vi "DynPid_filtered.vi"() -> ()   [LabVIEW 2019]
uses:
  <vilib>/Analysis/Matrix/Datatypes/RealMatrix.ctl
  <vilib>/userDefined/High Color/IMAQdx.ctl
  <vilib>/Platform/TimedLoop/XDataNode/timing_clust.ctl
  <vilib>/Platform/TimedLoop/XDataNode/nitl_modes.ctl
  <vilib>/Platform/TimedLoop/XDataNode/wakeup.ctl
  <vilib>/myRIO/Instrument Drivers/Onboard IO/AO/typedefs/AO Reference.ctl
  <vilib>/myRIO/Common/Instrument Driver Framework/Utilities/typedefs/myRIO Generic Hardware Reference.ctl
  <vilib>/myRIO/Common/Instrument Driver Framework/Utilities/typedefs/Hardware Version Enum.ctl
  <vilib>/myRIO/Common/Instrument Driver Framework/Utilities/typedefs/myRIO v1.0 Reference.ctl
  <vilib>/myRIO/Common/Instrument Driver Framework/Utilities/typedefs/Generic FPGA Reference.ctl
  <vilib>/myRIO/Common/Instrument Driver Framework/myRIO v1.0/AO/typedefs/AO Channels List.ctl
  <vilib>/myRIO/Common/Instrument Driver Framework/myRIO v1.0/AO/typedefs/AO Channels Enum.ctl
  <vilib>/myRIO/Common/Instrument Driver Framework/Utilities/typedefs/Analog Scaling Constants List.ctl
  <vilib>/myRIO/Common/Instrument Driver Framework/Utilities/typedefs/Analog Scaling Constants.ctl
  <vilib>/userDefined/High Color/nirio_resource_hc.ctl
  <vilib>/myRIO/Common/Instrument Driver Framework/myRIO v1.0/Encoder/typedefs/Encoder Signal Mode.ctl
  <vilib>/myRIO/Instrument Drivers/Onboard IO/Encoder/typedefs/Encoder Reference.ctl
  <vilib>/myRIO/Common/Instrument Driver Framework/myRIO v1.0/Encoder/typedefs/Encoder Channels Enum.ctl
  <vilib>/myRIO/Common/Instrument Driver Framework/myRIO v1.0/Encoder/typedefs/Encoder Configuration v1.0.ctl
  <vilib>/myRIO/Common/Instrument Driver Framework/Utilities/vis/Is FPGA Ref Available.vi
  <vilib>/myRIO/Common/Instrument Driver Framework/myRIO v1.0/AO/vis/myRIO v1.1 Open AO.vi
  <vilib>/myRIO/Instrument Drivers/Onboard IO/AO/vis/Write.vi
  <vilib>/myRIO/Common/Instrument Driver Framework/myRIO v1.0/Encoder/vis/myRIO v1.1 Open Encoder.vi
  <vilib>/myRIO/Instrument Drivers/Onboard IO/Encoder/vis/Read.vi
  <vilib>/myRIO/Common/Instrument Driver Framework/Utilities/vis/Validate Channels.vi
  <vilib>/myRIO/Common/Instrument Driver Framework/myRIO v1.0/AO/vis/myRIO v1.0 Reserve AO.vi
  <vilib>/myRIO/Common/Instrument Driver Framework/myRIO v1.0/Encoder/vis/myRIO v1.0 Reserve Encoder.vi
  <vilib>/Analysis/baseanly.llb/A x B.vi
  <vilib>/Analysis/baseanly.llb/A x Vector.vi
  <vilib>/myRIO/Common/Instrument Driver Framework/myRIO v1.0/AO/vis/myRIO v1.0 Build MUX Configuration AO.vi
  <vilib>/myRIO/Common/Instrument Driver Framework/myRIO v1.0/Resource Manager/vis/myRIO v1.0 Reserve Channel List.vi
  <vilib>/myRIO/Common/Instrument Driver Framework/myRIO v1.0/Encoder/vis/myRIO v1.0 Build MUX Configuration Encoder.vi
  <vilib>/myRIO/Common/Instrument Driver Framework/myRIO v1.0/Resource Manager/vis/myRIO v1.0 Reserve Channel.vi
  <vilib>/myRIO/Common/Instrument Driver Framework/myRIO v1.0/Resource Manager/vis/myRIO v1.0 Unreserve Channel.vi
  <vilib>/myRIO/Common/Instrument Driver Framework/myRIO v1.0/Resource Manager/vis/myRIO v1.0 Create Configuration List.vi
  <vilib>/myRIO/Common/Instrument Driver Framework/myRIO v1.0/Resource Manager/vis/myRIO v1.0 Build Mutex Name.vi
  <vilib>/Utility/VariantDataType/GetNumericInfo.vi
  <vilib>/Utility/error.llb/Error Cluster From Error Code.vi
  <vilib>/myRIO/Common/Instrument Driver Framework/myRIO v1.0/myRIO v1.1 Open.vi
  <vilib>/myRIO/Common/Instrument Driver Framework/myRIO v1.0/AO/vis/myRIO v1.0 Get Scaling Constants AO.vi
  <vilib>/myRIO/Common/Instrument Driver Framework/Utilities/vis/IO Manager.vi
  <vilib>/myRIO/Common/Instrument Driver Framework/Utilities/vis/Configuration Manager.vi
  <vilib>/myRIO/Common/Instrument Driver Framework/myRIO v1.0/myRIO v1.0 Close.vi
  <vilib>/myRIO/Common/Instrument Driver Framework/myRIO v1.0/AO/vis/myRIO v1.0 Write AO.vi
  <vilib>/Utility/file.llb/Write Delimited Spreadsheet (DBL).vi
  <vilib>/myRIO/Common/Instrument Driver Framework/myRIO v1.0/Resource Manager/vis/myRIO v1.0 Configure IO.vi
  <vilib>/myRIO/Common/Instrument Driver Framework/myRIO v1.0/Encoder/vis/myRIO v1.0 Configure Encoder.vi
  <vilib>/myRIO/Common/Instrument Driver Framework/myRIO v1.0/Encoder/vis/myRIO v1.0 Read Encoder.vi
  <vilib>/platform/TimedLoop/XDataNode/XDataNode.xnode
  <vilib>/myRIO/Express VI/Onboard IO/AO/AO Express VI.xnode
  <vilib>/myRIO/Instrument Drivers/Onboard IO/AO/vis/myRIO AO Open.xnode
  <vilib>/myRIO/Express VI/Onboard IO/Encoder/Encoder Express VI.xnode
  <vilib>/myRIO/Instrument Drivers/Onboard IO/Encoder/vis/myRIO Encoder Open.xnode
  <vilib>/myRIO/Common/Instrument Driver Framework/myRIO v1.0/Encoder/typedefs/Encoder Count Direction Enum.ctl
  <vilib>/Platform/TimedLoop/XDataNode/XDNodeRunTimeDep.lvlib
  <vilib>/myRIO/Instrument Drivers/Onboard IO/AO/AO.lvlib
  <vilib>/vision/driver/NI_Vision_Acquisition_Software.lvlib
  <vilib>/myRIO/Instrument Drivers/Onboard IO/Encoder/Encoder.lvlib
  <vilib>/vision/NI_Vision_Development_Module.lvlib
  <vilib>/Analysis/Matrix/NI_Matrix.lvlib
panel:
  out "ki_y":dbl
  out "kd_y":dbl
  out "kp_y":dbl
  out "ki_x":dbl
  out "kd_x":dbl
  out "kp_x":dbl
  out "scaled_obs_y":dbl[](array[numeric])
  out "scaled_obs_x":dbl[](array[numeric])
  out "done":bool
  out "target_y":dbl
  out "target_x":dbl
  in  "start_test":bool
  out "observation":dbl[](array[numeric])
  out "scaled_obs":dbl[](array[numeric])
  in  "record_name":string
  out "record":T1
  out "step_recorded":dbl
  in  "stop_recording":bool
  in  "start_recording":bool
  out "recording":bool
  out "record_t":dbl[](array[numeric])
  out "target_a_y":dbl(knob) scale=-45.0..45.0
  out "target_a_x":dbl(knob) scale=-45.0..45.0
  out "y_angle":dbl(knob) scale=-45.0..45.0
  out "x_angle":dbl(knob) scale=-45.0..45.0
  out "y_error":dbl
  out "x_error":dbl
  out "y":dbl
  out "x":dbl
  out "camera":T2(plugin-control)
  in  "threshold":cluster{"Lower value":sgl, "Upper value":sgl}={"Lower value"=60.0, "Upper value"=255.0} {"Upper value" format="%.2f"; "Lower value" format="%.2f"}
  out "threshold":T2(plugin-control)
  out "x-y":u32
  out "y_input":dbl
  out "y_angle_error":dbl
  out "x_angle_error":dbl
  in  "stop":bool
  out "x_input":dbl
  in  "reset":bool
  in  "dt":dbl=20.0
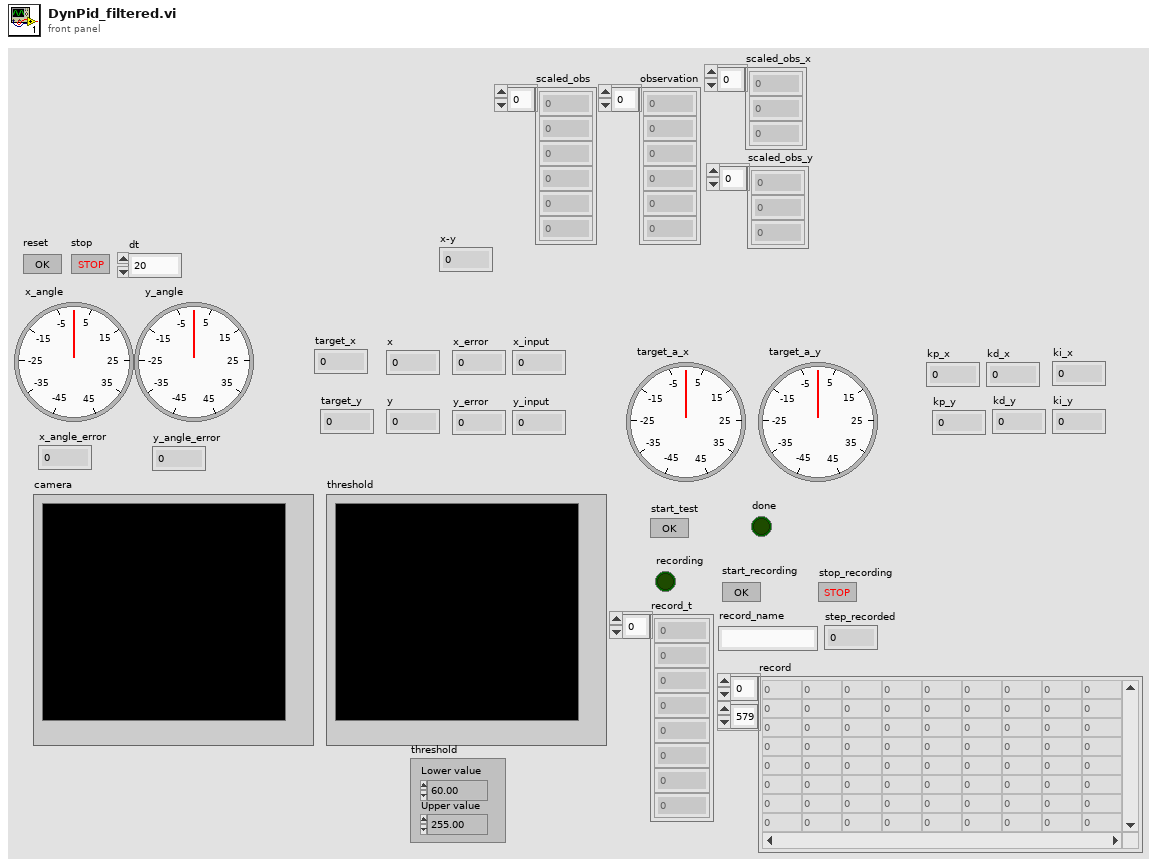
[diagram p1: front panel]
types:
  T1 = typedef "NI_Matrix.lvlib/RealMatrix.ctl" = dbl[][]
  T2 = typedef "IMAQ Image.ctl" = refnum<image>
  T3 = typedef "IMAQdx.ctl" = refnum<k21>
  T4 = typedef "XDNodeRunTimeDep.lvlib/timing_clust.ctl" = cluster{"Expected End [f-1]":u64, "Actual End [f-1]":u64, "Finished Late? [f-1]":bool, "Expected End [i-1]":u64, "Actual End [i-1]":u64, "Finished Late? [i-1]":bool, "Expected Start [i]":u64, "Actual Start [i]":u64, "Expected Start [f]":u64, "Actual Start [f]":u64, "Source Name":string, "Structure Name":string, "Period":i64, "Deadline":i64, "Offset":i64, "Start":i64, "Priority":i32, "Timeout":i32, "Mode":T5, "Wakeup Reason":T6, "Error":errorcluster, "Source Type":string, "Secondary Source Type":string, "Global End Time":u64, "Global Start Time":u64, "Frame Duration":u64, "Iteration Duration":u64, "Assigned CPU":i32, "I/O Scan Engine Mode":u32}
  T5 = typedef "XDNodeRunTimeDep.lvlib/nitl_modes.ctl" = enum32{"No Change", "Process missed periods, maintain original phase", "Discard missed periods, maintain original phase", "Process missed periods, ignore original phase", "Discard missed periods, ignore original phase"}
  T6 = typedef "XDNodeRunTimeDep.lvlib/wakeup.ctl" = enum32{"Normal", "Aborted", "Asynchronous wakeup", "Timing source error", "Timed loop error", "Timeout"}
  T7 = typedef "Encoder.lvlib/Encoder Reference.ctl" = cluster{"myRIO Reference":T8, "Encoder Channels Enum":T12}
  T8 = typedef "myRIO Generic Hardware Reference.ctl" = cluster{"myRIO Model":T9, "myRIO Hardware Reference":T10}
  T9 = typedef "Hardware Version Enum.ctl" = enum16{"Unknown", "myRIO-1900", "myRIO-1950", "roboRIO", "NI ELVIS RIO CM", "ELVIS III"}
  T10 = typedef "myRIO v1.0 Reference.ctl" = cluster{"Generic FPGA Reference":T11, "Allow multiple opens":bool}
  T11 = typedef "Generic FPGA Reference.ctl" = refnum<k20>
  T12 = typedef "Encoder Channels Enum.ctl" = enum16{"Not Connected", "C/ENC0", "C/ENC1", "A/ENC", "A/ENC0", "A/ENC1", "A/ENC2", "A/ENC3", "A/ENC4", "A/ENC5", "A/ENC6", "A/ENC7", "A/ENC8", "A/ENC9", "B/ENC", "B/ENC0", "B/ENC1", "B/ENC2", "B/ENC3", "B/ENC4", "B/ENC5", "B/ENC6", "B/ENC7", "B/ENC8", "B/ENC9", "DIO/ENC0", "DIO/ENC1", "DIO/ENC2", "DIO/ENC3", "DIO/ENC4"}
  T13 = typedef "Encoder Signal Mode.ctl" = enum16{"Quadrature phase signal", "Step and direction signal"}
  T14 = typedef "nirio_resource_hc.ctl" = tag
  T15 = typedef "AO.lvlib/AO Reference.ctl" = cluster{"myRIO Reference":T8, "AO Channel List":T16, "AO Scaling Constant List":T18}
  T16 = typedef "AO Channels List.ctl" = T17[]
  T17 = typedef "AO Channels Enum.ctl" = enum16{"Not Connected", "AudioOut/Left", "AudioOut/Right", "C/AO0", "C/AO1", "A/AO0", "A/AO1", "B/AO0", "B/AO1"}
  T18 = typedef "Analog Scaling Constants List.ctl" = T19[]
  T19 = typedef "Analog Scaling Constants.ctl" = cluster{"LSB Weight (Volts)":dbl, "Offset (Volts)":dbl, "Signed?":bool}
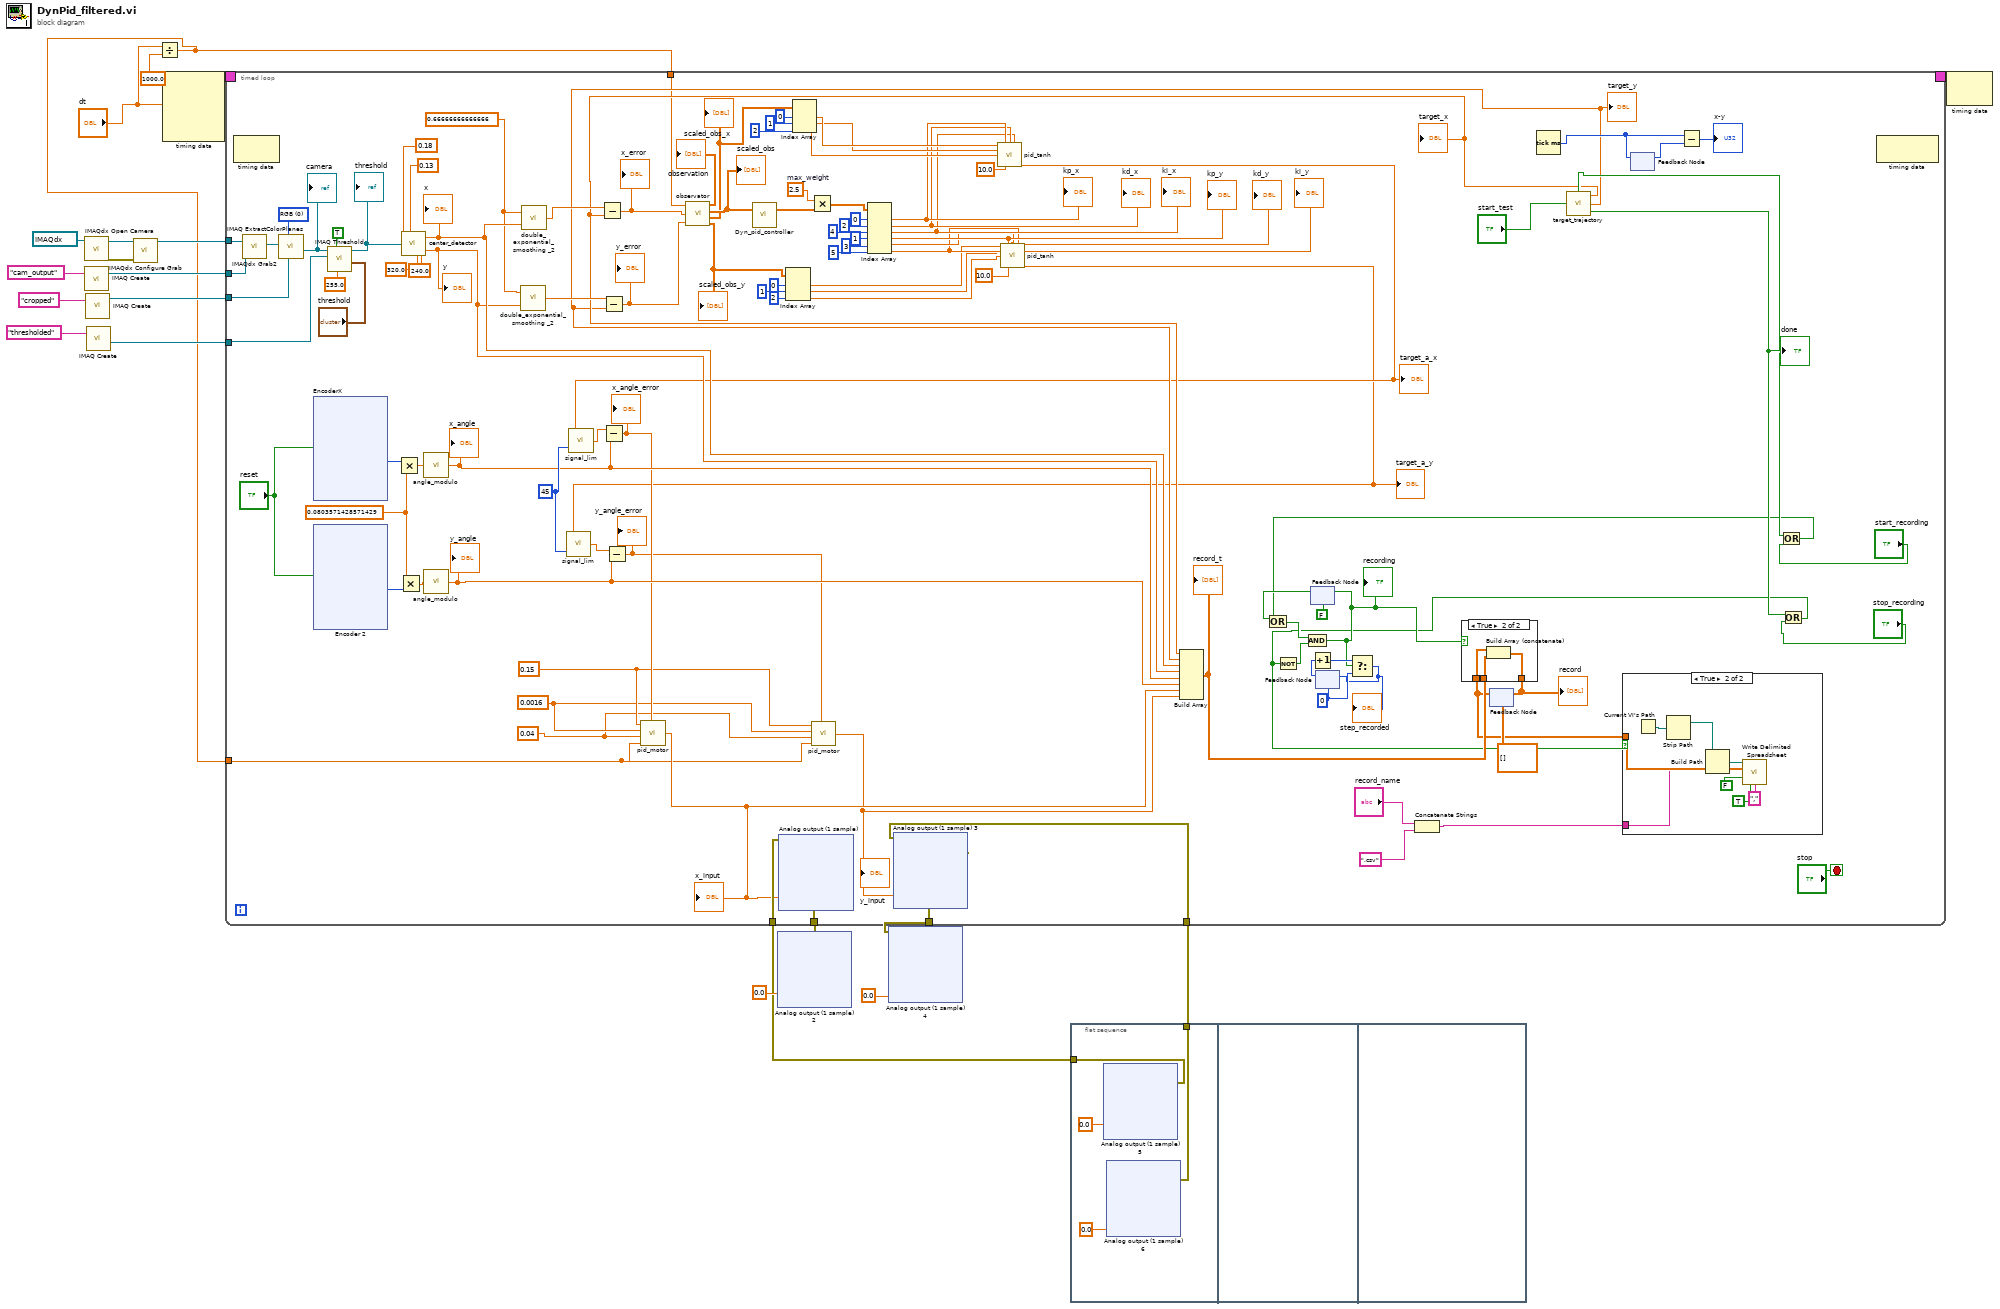
[diagram p0: block diagram]
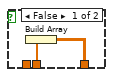
[diagram p3: hidden frame]
diagram:
  n1 = call <vilib>:"IMAQdx Open Camera.vi"("Session In"=T3 "cam2") -> ("error out"=w13:errorcluster, "Session Out"=w14:T3)  [unwired: 9 in]
  n2 = call "IMAQ Create"("Image Name"="cam_output") -> ("New Image"=w15:T2)  [unwired: 4 in, 1 out]
  n3 = call "IMAQ Create"("Image Name"="cropped") -> ("New Image"=w6:T2)  [unwired: 4 in, 1 out]
  n4 = call "IMAQ Create"("Image Name"="thresholded") -> ("New Image"=w4:T2)  [unwired: 4 in, 1 out]
  n5 = call <vilib>:"IMAQdx Configure Grab.vi"("error in"=w13, "Session In"=w14) -> ("Session Out"=w16:T3)  [unwired: 8 in, 1 out]
  n6 = Divide(x="dt", y=1000.0) -> (x/y=w1:dbl)
  n7 = node-c288("dt") -> (w21:T4)  [unwired: 3 in]
  n8 = timed-loop {
    timing: w21 -> [_]
    timing-out: [_] -> w20
    tunnel: w16 -> [w131]
    tunnel: w15 -> [w130]
    tunnel: w1 -> [w72]
    tunnel: [w119] -> w11
    tunnel: [w115] -> w10
    tunnel: w9 -> [w114]
    tunnel: w8 -> [w113]
    tunnel: w6 -> [w88]
    tunnel: w4 -> [w82]
    tunnel: w1 -> [w60]
    stop <- "stop" stop-if-true
    w24 = 2.5  # max_weight
    w77 = 0.66666666666666
    w69 = 0.04 ("ki")
    w70 = 0.0016 ("kd")
    w71 = 0.15 ("kp")
    w91 = u16 0 items=["RGB", "HSL", "HSV", "HSI"] ("Color Mode")
    w101 = 0
    w120 = 45
    w128 = 0.0803571428571429
    n9 = node-c288() -> ()  [unwired: 1 in, 1 out]
    n10 = call <vilib>:"IMAQdx Grab2.vi"("Image In"=w130, "Session In"=w131) -> ("Image Out"=w90:T2)  [unwired: 6 in, 3 out]
    n11 = call "IMAQ ExtractColorPlanes"("Blue or Luma or Val or Inten Plane"=w88, "Color Mode"=w91, "Image Src"=w90) -> ("Blue or Luma or Val or Inten Plane out"=w89:T2)  [unwired: 5 in, 3 out]
    "camera" <- w89
    n12 = xnode "EncoderX"("Reset Counter"="reset") -> ("Counter Value"=w129:i32)  [unwired: 1 in, 3 out]
    n13 = xnode "Encoder 2"("Reset Counter"="reset") -> ("Counter Value"=w127:i32)  [unwired: 1 in, 3 out]
    n14 = call "IMAQ Threshold"("Replace Value"=sgl 255.0, "Keep/Replace Value (Replace)"=TRUE, "Range"="threshold", "Image Dst"=w82, "Image Src"=w89) -> ("Image Dst Out"=w85:T2)  [unwired: 5 in, 1 out]
    "threshold" <- w85
    n15 = Multiply(x=w129, y=w128) -> (x*y=w124:dbl)
    n16 = Multiply(x=w128, y=w127) -> (x*y=w123:dbl)
    n17 = call "center_detector.vi"("px_x"=320.0, "px_y"=240.0, "Image"=w85, "m_x"=0.18, "m_y"=0.13) -> ("x"=w80:dbl, "y"=w78:dbl)
    "x" <- w80
    "y" <- w78
    n18 = call "angle_modulo.vi"("alpha"=w124) -> ("alpha_prime"=w109:dbl)
    "x_angle" <- w109
    n19 = call "angle_modulo.vi"("alpha"=w123) -> ("alpha_prime"=w108:dbl)
    "y_angle" <- w108
    n20 = call "double_exponential_smoothing _2.vi"("x"=w78, "alpha"=w77) -> ("dema"=w79:dbl)
    n21 = call "double_exponential_smoothing _2.vi"("x"=w80, "alpha"=w77) -> ("dema"=w81:dbl)
    n22 = feedback #1(FALSE) -> (w107:bool)
    n23 = feedback #2(w101) -> (w103:i32)
    n24 = Increment(x=w103) -> (x+1=w102:i32)
    n25 = Concatenate Strings("record_name", ".csv") -> (w92:string)
    n26 = feedback #3(T1 [] ("Real Matrix")) -> (w95:T1)
    n27 = Tick Count (ms)() -> (millisecond timer value=w118:u32)
    n28 = call "target_trajectory.vi"("start_test"="start_test") -> ("start"=w65:bool, "target_x"=w62:dbl, "target_y"=w61:dbl, "done"=w66:bool)
    "target_x" <- w62
    "target_y" <- w61
    "done" <- w66
    n29 = Subtract(x=w81, y=w62) -> (x-y=w59:dbl)
    "x_error" <- w59
    n30 = Subtract(x=w79, y=w61) -> (x-y=w58:dbl)
    "y_error" <- w58
    n31 = call "observator.vi"("d_t"=w60, "e_x"=w59, "e_y"=w58) -> ("observation"=→"observation":dbl[], "scaled_obs"=w55:dbl[], "scaled_obs_x"=w48:dbl[], "scaled_obs_y"=w44:dbl[])
    "scaled_obs" <- w55
    "scaled_obs_x" <- w48
    "scaled_obs_y" <- w44
    n32 = call "Dyn_pid_controller.vi"("Normalized observation"=w55) -> ("output"=w23:dbl[])  [unwired: 1 in, 1 out]
    n33 = Index Array(array=w44, index #1=0 ("index"), index #2=1 ("index"), index #3=2 ("index")) -> (element #1=w29:dbl, element #2=w28:dbl, element #3=w27:dbl)
    n34 = Index Array(array=w48, index #1=0 ("index"), index #2=1 ("index"), index #3=2 ("index")) -> (element #1=w40:dbl, element #2=w39:dbl, element #3=w38:dbl)
    n35 = Multiply(x=w24, y=w23) -> (x*y=w22:dbl[])
    n36 = Index Array(array=w22, index #1=0 ("index"), index #2=2 ("index"), index #3=4 ("index"), index #4=1 ("index"), index #5=3 ("index"), index #6=5 ("index")) -> (element #1=w37:dbl, element #2=w36:dbl, element #3=w35:dbl, element #4=w32:dbl, element #5=w31:dbl, element #6=w30:dbl)
    "kp_x" <- w37
    "kd_x" <- w36
    "ki_x" <- w35
    "kp_y" <- w32
    "kd_y" <- w31
    "ki_y" <- w30
    n37 = call "pid_tanh.vi"("err"=w40, "kp"=w37, "kd"=w36, "ki"=w35, "d_err"=w39, "i_error"=w38, "max_u"=10.0) -> ("u"=w33:dbl)  [unwired: 8 in]
    "target_a_x" <- w33
    n38 = call "signal_lim.vi"("lim"=w120, "x"=w33) -> ("y"=w122:dbl)
    n39 = Subtract(x=w122, y=w109) -> (x-y=w76:dbl)
    "x_angle_error" <- w76
    n40 = call "pid_motor.vi"("kp"=w71, "kd"=w70, "ki"=w69, "dt"=w72, "err"=w76) -> ("u"=w75:dbl)
    "x_input" <- w75
    n41 = xnode "Analog output (1 sample)"("C/AO0 (AO0)"=w75, "error in (no error)"=w114) -> ("error out"=w119:errorcluster)
    n42 = call "pid_tanh.vi"("err"=w29, "kp"=w32, "kd"=w31, "ki"=w30, "d_err"=w28, "i_error"=w27, "max_u"=10.0) -> ("u"=w25:dbl)  [unwired: 8 in]
    "target_a_y" <- w25
    n43 = call "signal_lim.vi"("lim"=w120, "x"=w25) -> ("y"=w121:dbl)
    n44 = Subtract(x=w121, y=w108) -> (x-y=w74:dbl)
    "y_angle_error" <- w74
    n45 = call "pid_motor.vi"("kp"=w71, "kd"=w70, "ki"=w69, "dt"=w72, "err"=w74) -> ("u"=w73:dbl)
    "y_input" <- w73
    n46 = xnode "Analog output (1 sample) 3"("C/AO1 (AO1)"=w73, "error in (no error)"=w113) -> ("error out"=w115:errorcluster)
    n47 = Build Array(w62, w61, w80, w78, w109, w108, w75, w73) -> (w98:dbl[])
    "record_t" <- w98
    n48 = feedback-in #4(w118) -> ()
    n49 = feedback #4() -> (w117:u32)  [unwired: 1 in]
    n50 = Subtract(x=w118, y=w117) -> (x-y=→"x-y":u32)
    n51 = Or(x=w65, y="start_recording") -> (x .or. y?=w64:bool)
    n52 = Or(x=w107, y=w64) -> (x .or. y?=w106:bool)
    n53 = Or(x=w66, y="stop_recording") -> (x .or. y?=w56:bool)
    n54 = Not(x=w56) -> (.not. x?=w105:bool)
    n55 = And(x=w106, y=w105) -> (x .and. y?=w99:bool)
    "recording" <- w99
    n56 = feedback-in #1(w99) -> ()
    n57 = Select(t=w102, s=w99, f=w101) -> (s? t:f=w100:i32)
    "step_recorded" <- w100
    n58 = feedback-in #2(w100) -> ()
    n59 = case shown="True" w99 {
      tunnel: w95 -> [_ w144]
      tunnel: [w140 w143] -> w96
      tunnel: w98 -> [w141 w142]
      frame False {
        n60 = Build Array(w141) -> (w140:T1)
      }
      frame True {
        n61 = Build Array (concatenate)(w144, w142) -> (w143:T1)
      }
    }
    "record" <- w96
    n62 = feedback-in #3(w96) -> ()
    n63 = case shown="True" w56 {
      tunnel: w95 -> [_ w139]
      tunnel: w92 -> [_ w137]
      frame False {
      }
      frame True {
        n64 = Current VI's Path() -> (path=w135:path)
        n65 = Strip Path(path=w135) -> (stripped path=w134:path)  [unwired: 1 out]
        n66 = Build Path(base path=w134, name or relative path=w137) -> (appended path=w136:path)
        n67 = call-poly <vilib>:"Write Delimited Spreadsheet.vi"("file path (dialog if empty)"=w136, "2D data"=w139, "append to file? (new file:F)"=FALSE, "transpose? (no:F)"=TRUE, "delimiter (\\t)"="," ("delimiter (\\t)")) -> ()  [unwired: 9 in, 2 out]
      }
    }
    n68 = node-c288() -> ()  [unwired: 1 in, 1 out]
  }
  n69 = xnode "Analog output (1 sample) 2"("C/AO0 (AO0)"=0.0, "error in (no error)"=w11) -> ()  [unwired: 1 out]
  n70 = xnode "Analog output (1 sample) 4"("C/AO1 (AO1)"=0.0, "error in (no error)"=w10) -> ()  [unwired: 1 out]
  n71 = flat-sequence {
    tunnel: [w314] -> w9
    tunnel: [w313] -> w8
    frame #0 {
      n72 = xnode "Analog output (1 sample) 5"("C/AO0 (AO0)"=0.0) -> ("error out"=w314:errorcluster)  [unwired: 1 in]
      n73 = xnode "Analog output (1 sample) 6"("C/AO1 (AO1)"=0.0) -> ("error out"=w313:errorcluster)  [unwired: 1 in]
    }
    frame #1 {
    }
    frame #2 {
    }
  }
  n74 = node-c288(w20) -> ()  [unwired: 1 out]
